vi "sub_inverse_kin6.vi"(1 "Manipulator calibration":T2={"Tool offsets"=[], "Handle light calibration"=[], "Base pivots"=[], "Output pivots"=[], "Length center"=0.0, "Workspace height"=[], "Workspace diameter"=[0.0, 0.0, 36200.0], "Stack travel"=400.0, "Saturation pos"=375.0, "Inverse filters"=[], "Strut length"=0.0} {"Strut length" format="%#_4p"; "Saturation pos" format="%#.1f"; "Stack travel" format="%#.1f"; "Length center" format="%#_4p"; "Output pivots" format="%#_6f"; "Base pivots" format="%#_6f"; "Handle light calibration" format="%#.1f"}, 2 "Output pivots":sgl[][](array[numeric]), 3 "Transform":T1) -> (0 "Link lengths":sgl[](array[numeric]))   [LabVIEW 2014]
uses:
  testing/manipulator_cal.ctl
  asap/labview/testing/probe_calibration.ctl
  <vilib>/Analysis/Matrix/Datatypes/RealMatrix.ctl
  <vilib>/Analysis/baseanly.llb/A x Vector.vi
  <vilib>/Analysis/NI_AALBase.lvlib
  <vilib>/Analysis/Matrix/NI_Matrix.lvlib
panel:
  # "Find link lengths given output pivots and transform that converts the output pivots into handle coordinates."
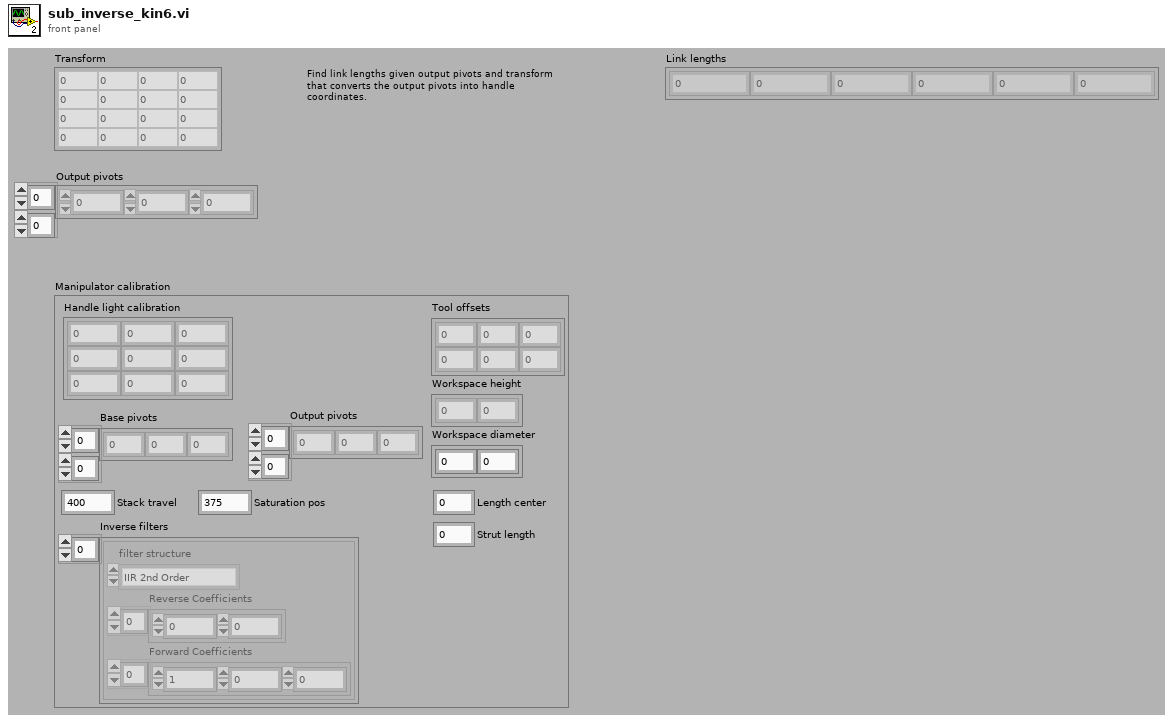
[diagram p1: front panel]
types:
  T1 = typedef "NI_Matrix.lvlib/RealMatrix.ctl" = dbl[][]
  T2 = typedef "manipulator_cal.ctl" = cluster{"Tool offsets":sgl[][], "Handle light calibration":T3, "Base pivots":sgl[][], "Output pivots":sgl[][], "Length center":sgl, "Workspace height":sgl[], "Workspace diameter":sgl[], "Stack travel":sgl, "Saturation pos":sgl, "Inverse filters":cluster{"filter structure":enum32{"IIR 2nd Order", "IIR 4th Order"}, "Reverse Coefficients":dbl[], "Forward Coefficients":dbl[]}[], "Strut length":sgl}
  T3 = typedef "probe_calibration.ctl" = sgl[][]
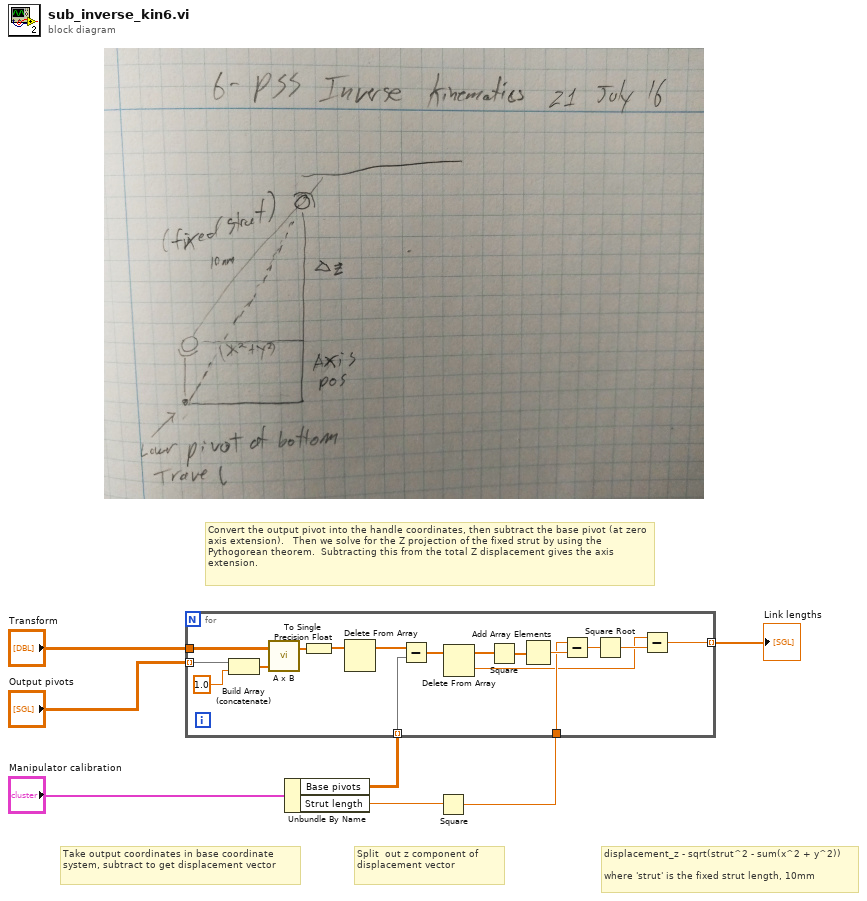
[diagram p0: block diagram]
diagram:
  # "displacement_z - sqrt(strut^2 - sum(x^2 + y^2))\n\nwhere 'strut' is the fixed strut length, 10mm"
  # "Split  out z component of displacement vector"
  # "Take output coordinates in base coordinate system, subtract to get displacement vector"
  # "Convert the output pivot into the handle coordinates, then subtract the base pivot (at zero axis extension).   Then we solve for the Z projection of the fixed strut by using the Pythogorean theorem.  Subtracting this from the total Z displacement gives the axis extension."
  n1 = Unbundle By Name("Manipulator calibration") -> ("Base pivots"=w4:sgl[][], "Strut length"=w2:sgl)
  n2 = Square(x=w2) -> (x^2=w1:sgl)
  n3 = for {
    tunnel: "Output pivots" -> [w20] mode=indexing
    tunnel: "Transform" -> [w19]
    tunnel: w4 -> [w17] mode=indexing
    tunnel: [w8] -> w5 mode=indexing
    tunnel: w1 -> [w15]
    n4 = Build Array (concatenate)(w20, sgl 1.0) -> (w23:sgl[])
    n5 = call-poly <vilib>:"A x B.vi"("Vector"=w23, "A"=w19) -> ("A x Vector"=w21:dbl[])  [unwired: 1 out]
    n6 = To Single Precision Float(number=w21) -> (single precision float=w24:sgl[])
    n7 = Delete From Array(array=w24) -> (array with subset deleted=w18:sgl[])  [unwired: 2 in, 1 out]
    n8 = Subtract(x=w18, y=w17) -> (x-y=w11:sgl[])
    n9 = Delete From Array(array=w11) -> (deleted portion=w12:sgl, array with subset deleted=w10:sgl[])  [unwired: 2 in]
    n10 = Square(x=w10) -> (x^2=w9:sgl[])
    n11 = Add Array Elements(numeric array=w9) -> (sum=w16:sgl)
    n12 = Subtract(x=w15, y=w16) -> (x-y=w14:sgl)
    n13 = Square Root(x=w14) -> (sqrt(x)=w13:sgl)
    n14 = Subtract(x=w12, y=w13) -> (x-y=w8:sgl)
  }
  "Link lengths" <- w5
